vi "Decimal_point.vi"(11 "Numeric":dbl format="%.3f") -> (0 "2|3?":bool, 3 "Decimal?":bool, 6 "1|2?":bool)   [LabVIEW 2020]
panel:
  out "x*y":dbl format="%.6f"
  out "x-y*floor(x/y)":dbl
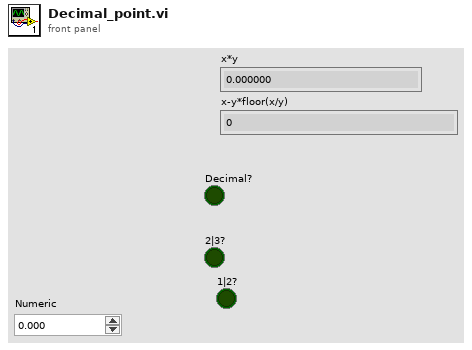
[diagram p1: front panel]
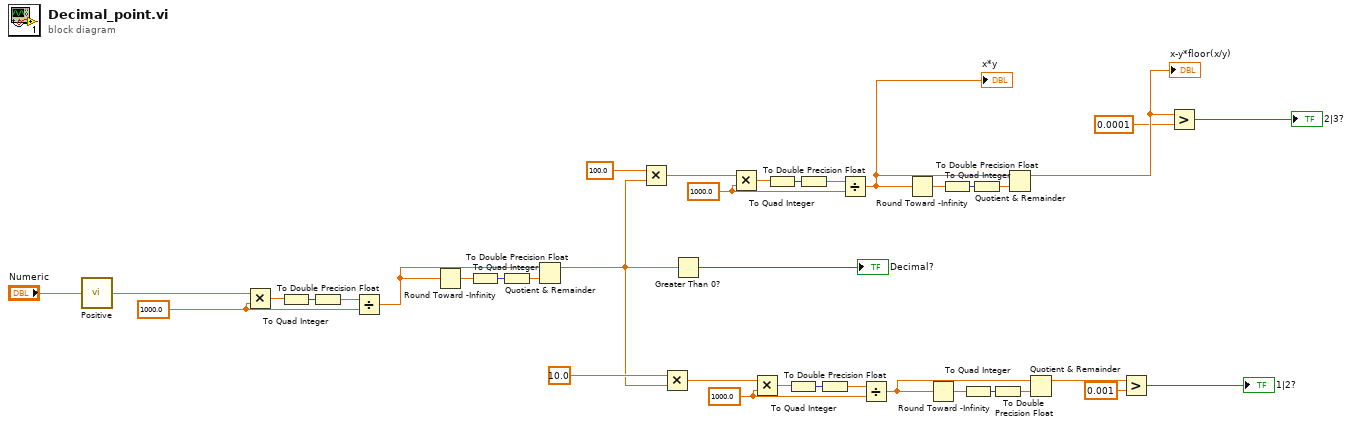
[diagram p0: block diagram]
diagram:
  w10 = 1000.0 ("y")
  w19 = 1000.0 ("y")
  w26 = 1000.0 ("y")
  n1 = call <userlib>:"Positive.vi"("In"="Numeric") -> ("Out"=w21:dbl)  [unwired: 6 in]
  n2 = Multiply(x=w21, y=w26) -> (x*y=w28:dbl)
  n3 = To Quad Integer(1:w28) -> (0:w27:i64)
  n4 = To Double Precision Float(number=w27) -> (double precision float=w25:dbl)
  n5 = Divide(x=w25, y=w26) -> (x/y=w23:dbl)
  n6 = Round Toward -Infinity(1:w23) -> (0:w38:dbl)
  n7 = To Quad Integer(1:w38) -> (0:w37:i64)
  n8 = To Double Precision Float(number=w37) -> (double precision float=w36:dbl)
  n9 = Quotient & Remainder(x=w23, y=w36) -> (x-y*floor(x/y)=w4:dbl)  [unwired: 1 out]
  n10 = Multiply(x=100.0, y=w4) -> (x*y=w16:dbl)
  n11 = Multiply(x=10.0, y=w4) -> (x*y=w13:dbl)
  n12 = Greater Than 0?(x=w4) -> (x > 0?=→"Decimal?":bool)
  n13 = Multiply(x=w16, y=w19) -> (x*y=w17:dbl)
  n14 = Multiply(x=w13, y=w10) -> (x*y=w12:dbl)
  n15 = To Quad Integer(1:w17) -> (0:w18:i64)
  n16 = To Quad Integer(1:w12) -> (0:w11:i64)
  n17 = To Double Precision Float(number=w18) -> (double precision float=w20:dbl)
  n18 = To Double Precision Float(number=w11) -> (double precision float=w9:dbl)
  n19 = Divide(x=w20, y=w19) -> (x/y=w15:dbl)
  "x*y" <- w15
  n20 = Divide(x=w9, y=w10) -> (x/y=w14:dbl)
  n21 = Round Toward -Infinity(1:w15) -> (0:w32:dbl)
  n22 = Round Toward -Infinity(1:w14) -> (0:w7:dbl)
  n23 = To Quad Integer(1:w32) -> (0:w33:i64)
  n24 = To Quad Integer(1:w7) -> (0:w6:i64)
  n25 = To Double Precision Float(number=w33) -> (double precision float=w34:dbl)
  n26 = To Double Precision Float(number=w6) -> (double precision float=w5:dbl)
  n27 = Quotient & Remainder(x=w15, y=w34) -> (x-y*floor(x/y)=w29:dbl)  [unwired: 1 out]
  "x-y*floor(x/y)" <- w29
  n28 = Quotient & Remainder(x=w14, y=w5) -> (x-y*floor(x/y)=w1:dbl)  [unwired: 1 out]
  n29 = Greater?(x=w1, y=0.001 ("x")) -> (0:→"1|2?":bool)
  n30 = Greater?(x=w29, y=0.0001 ("x")) -> (0:→"2|3?":bool)
